vi "数字键盘.vi"(1 "OldNumber":sgl) -> (0 "NewNumber":sgl)   [LabVIEW 2016, in "中水三立SQL数据传输.lvlib"]
panel:
  in  "数值":dbl
  in  "OK Button":bool
  in  "Cancel":bool
  in  "OK":bool
  in  "Clear":bool
  in  "BackSpace":bool
  in  "String":string
  in  "Point":bool
  in  "Zero":bool
  in  "Nine":bool
  in  "Eight":bool
  in  "Seven":bool
  in  "Six":bool
  in  "Five":bool
  in  "Four":bool
  in  "Three":bool
  in  "Two":bool
  in  "One":bool
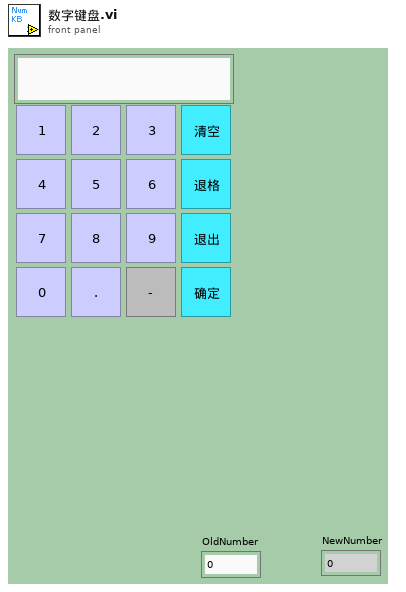
[diagram p1: front panel]
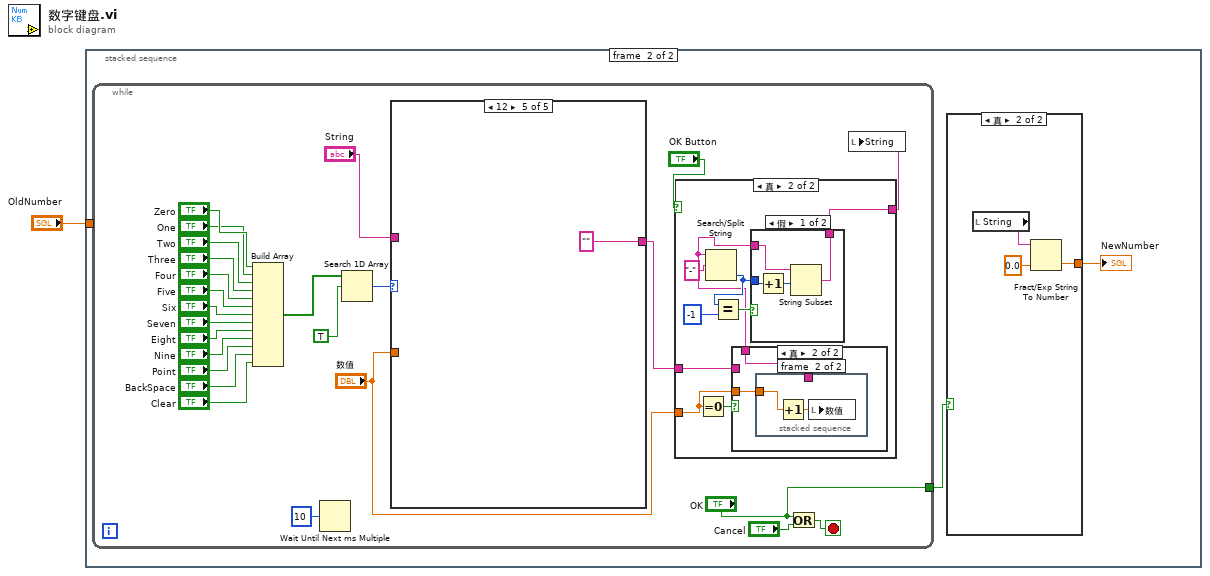
[diagram p0: block diagram]
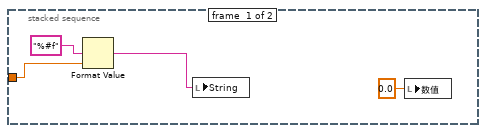
[diagram p2: hidden frame]
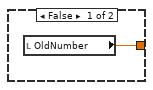
[diagram p3: hidden frame]
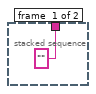
[diagram p6: hidden frame]
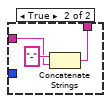
[diagram p7: hidden frame]
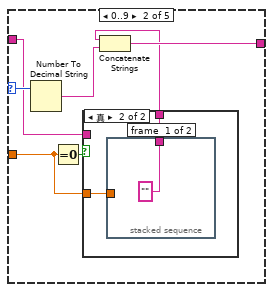
[diagram p9: hidden frame]
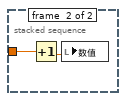
[diagram p11: hidden frame]
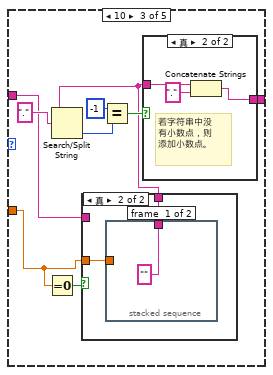
[diagram p12: hidden frame]
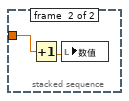
[diagram p14: hidden frame]
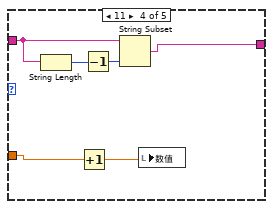
[diagram p16: hidden frame]
diagram:
  n1 = stacked-sequence {
    tunnel: "OldNumber" -> [w2 _]
    frame #0 {
      n2 = Format Value(format string="%#f" ("格式字符串"), value (0)=w2) -> (output string=w3:string)  [unwired: 1 in]
      n3 = local write "String"(w3) -> ()
      n4 = local write "数值"(0.0 ("数值")) -> ()
    }
    frame #1 {
      n5 = while {
        tunnel: ["OK"] -> w7
        stop <- w35 stop-if-true
        n6 = Build Array("Zero", "One", "Two", "Three", "Four", "Five", "Six", "Seven", "Eight", "Nine", "Point", "BackSpace", "Clear") -> (w20:bool[])
        n7 = Wait Until Next ms Multiple(millisecond multiple=u32 10) -> ()  [unwired: 1 out]
        n8 = Search 1D Array(1D array=w20, element=TRUE) -> (index of element=w18:i32)  [unwired: 1 in]
        n9 = case shown="12" w18 {
          selector: w18 -> [_ w67 _ _ _]
          tunnel: "String" -> [w60 w62 w77 w97 _]
          tunnel: [w60 w65 w78 w95 "" ("String")] -> w12
          tunnel: "数值" -> [_ w61 w74 w94 _]
          frame Default {
          }
          frame 0..9 {
            n10 = Number To Decimal String(number=w67) -> (decimal integer string=w66:string)  [unwired: 1 in]
            n11 = Equal To 0?(x=w61) -> (x = 0?=w64:bool)
            n12 = case shown="真" w64 {
              tunnel: [w68 w70] -> w63
              tunnel: w61 -> [_ w69]
              tunnel: w62 -> [w68 _]
              frame False {
              }
              frame True {
                n13 = stacked-sequence {
                  tunnel: ["" _] -> w70
                  tunnel: w69 -> [_ w73]
                  frame #0 {
                  }
                  frame #1 {
                    n14 = Increment(x=w73) -> (x+1=w72:dbl)
                    n15 = local write "数值"(w72) -> ()
                  }
                }
              }
            }
            n16 = Concatenate Strings(w63, w66) -> (w65:string)
          }
          frame 10 {
            n17 = Equal To 0?(x=w74) -> (x = 0?=w76:bool)
            n18 = case shown="真" w76 {
              tunnel: [w83 w85] -> w75
              tunnel: w77 -> [w83 _]
              tunnel: w74 -> [_ w84]
              frame False {
              }
              frame True {
                n19 = stacked-sequence {
                  tunnel: ["" _] -> w85
                  tunnel: w84 -> [_ w87]
                  frame #0 {
                  }
                  frame #1 {
                    n20 = Increment(x=w87) -> (x+1=w88:dbl)
                    n21 = local write "数值"(w88) -> ()
                  }
                }
              }
            }
            n22 = Search/Split String(string=w75, search string/char (-)=".") -> (offset of match=w81:i32)  [unwired: 1 in, 2 out]
            n23 = Equal?(x=-1, y=w81) -> (x = y?=w79:bool)
            n24 = case shown="真" w79 {
              tunnel: w75 -> [w89 w92]
              tunnel: [w89 w90] -> w78
              frame False {
              }
              frame True {
                # "若字符串中没\n有小数点，则\n添加小数点。"
                n25 = Concatenate Strings(w92, "." ("string")) -> (w90:string)
              }
            }
          }
          frame 11 {
            n26 = String Length(string=w97) -> (length=w96:i32)
            n27 = Increment(x=w94) -> (x+1=w93:dbl)
            n28 = Decrement(x=w96) -> (x-1=w98:i32)
            n29 = String Subset(string=w97, length (rest)=w98) -> (substring=w95:string)  [unwired: 1 in]
            n30 = local write "数值"(w93) -> ()
          }
          frame 12 {
          }
        }
        n31 = case shown="真" "OK Button" {
          tunnel: [w37 w43] -> w15
          tunnel: "数值" -> [_ w40]
          tunnel: w12 -> [w37 w39]
          frame False {
          }
          frame True {
            n32 = Equal To 0?(x=w40) -> (x = 0?=w41:bool)
            n33 = case shown="真" w41 {
              tunnel: [w47 w49] -> w38
              tunnel: w40 -> [_ w48]
              tunnel: w39 -> [w47 _]
              frame False {
              }
              frame True {
                n34 = stacked-sequence {
                  tunnel: ["" _] -> w49
                  tunnel: w48 -> [_ w51]
                  frame #0 {
                  }
                  frame #1 {
                    n35 = Increment(x=w51) -> (x+1=w52:dbl)
                    n36 = local write "数值"(w52) -> ()
                  }
                }
              }
            }
            n37 = Search/Split String(string=w38, search string/char (-)="-" ("搜索字符串/字符(-)")) -> (offset of match=w42:i32)  [unwired: 1 in, 2 out]
            n38 = Equal?(x=w42, y=-1) -> (x = y?=w44:bool)
            n39 = case shown="假" w44 {
              tunnel: w38 -> [w56 w58]
              tunnel: [w55 w57] -> w43
              tunnel: w42 -> [w54 _]
              frame False {
                n40 = Increment(x=w54) -> (x+1=w53:i32)
                n41 = String Subset(string=w56, offset (0)=w53) -> (substring=w55:string)  [unwired: 1 in]
              }
              frame True {
                n42 = Concatenate Strings("-" ("string"), w58) -> (w57:string)
              }
            }
          }
        }
        n43 = Or(x="OK", y="Cancel") -> (x .or. y?=w35:bool)
        n44 = local write "String"(w15) -> ()
      }
      n45 = case shown="真" w7 {
        tunnel: [w8 w9] -> w6
        frame False {
          n46 = local read "OldNumber"() -> (w8:sgl)
        }
        frame True {
          n47 = local read "String"() -> (w11:string)
          n48 = Fract/Exp String To Number(string=w11, default (0 dbl)=sgl 0.0 ("default (0 DBL)")) -> (number=w9:sgl)  [unwired: 2 in, 1 out]
        }
      }
      "NewNumber" <- w6
    }
  }
